vi "Original Config.vi"(11 "Config File":refnum<class "JSONConfigFile.lvclass">) -> (2 "Original Config (as read from the file)":string="{}")   [LabVIEW 2021, in "json.facade.lvlib" / "JSONConfigFile.lvclass"]
doc: "The original config info as initially read from the config file (as as most recently written by this Config File object)."
uses:
  JSONConfigFile.lvclass
  JSONConfigFile.lvclass/JSONConfigFile.ctl
  jsontext/Config Files/Config File.lvclass
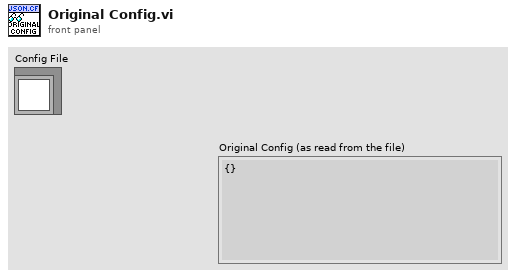
[diagram p1: front panel]
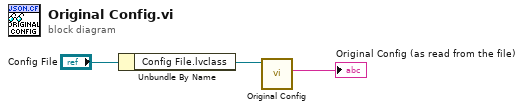
[diagram p0: block diagram]
diagram:
  n1 = Unbundle By Name("Config File") -> ("Config File.lvclass"=w1:refnum<class "Config File.lvclass">)
  n2 = call "Original Config.vi"("Config File in"=w1) -> ("Original Config (as read from the file)"=→"Original Config (as read from the file)":string)  [unwired: 10 in]
